vi "start_visa.vi"() -> (3 "output cluster":T1)   [LabVIEW 2020]
uses:
  <vilib>/Instr/_visa.llb/VISA Find Search Mode.ctl
  <vilib>/Instr/_visa.llb/VISA Configure Serial Port (Instr).vi
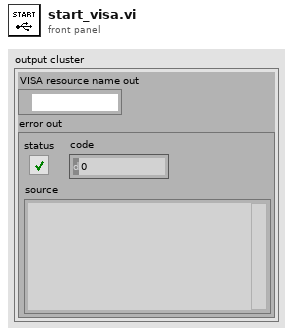
[diagram p1: front panel]
types:
  T1 = cluster{"VISA resource name out":refnum<visa-resource-name>, "error out":errorcluster}
  T2 = typedef "VISA Find Search Mode.ctl" = u32
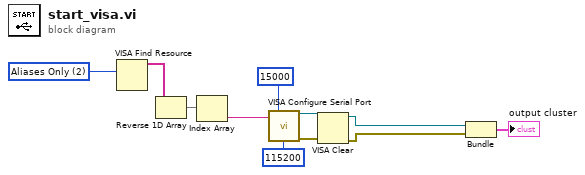
[diagram p0: block diagram]
diagram:
  w11 = T2 2 items=["Canonical Names Only"=0, "Aliases Only"=2, "Include Matching Aliases"=3, "Include All Aliases"=4] ("Search Mode")
  n1 = VISA Find Resource(10:w11) -> (3:w9:string[])  [unwired: 2 in, 2 out]
  n2 = Reverse 1D Array(array=w9) -> (reversed array=w10:string[])
  n3 = Index Array "Index Array"(array=w10) -> (element=w4:string)  [unwired: 1 in]
  n4 = call-poly "VISA Configure Serial Port"("VISA resource name"=w4, "timeout (10sec)"=u32 15000, "baud rate (9600)"=u32 115200) -> ("VISA resource name out"=w5:refnum<visa-resource-name>, "error out"=w6:errorcluster)  [unwired: 11 in]
  n5 = VISA Clear(VISA resource name=w5, error in (no error)=w6) -> (VISA resource name out=w2:refnum<visa-resource-name>, error out=w1:errorcluster)
  n6 = Bundle("VISA resource name out"=w2, "error out"=w1) -> (→"output cluster":T1)  [unwired: 1 in]
